vi "Zaber Manager.vi"(0 "Cmd":string="192.168.33.1", 1 "Action":T1=enum."Init", 5 "Value":dbl, 7 "File Path":path, 11 "error in (no error)":errorcluster) -> (4 "Response":string, 6 "Connected":bool, 8 "Position(um)":dbl, 10 "Position(cnts)":i64, 13 "Success":bool, 14 "Timeout":bool, 15 "error out":errorcluster)   [LabVIEW 2020]
uses:
  Mot Stage Mngr.ctl
  Lib/Serial/Find Device Protocols.ctl
  Hardware Globals.vi
  Zaber/Zaber A Series.lvlib
  Lib/Utilities.lvlib
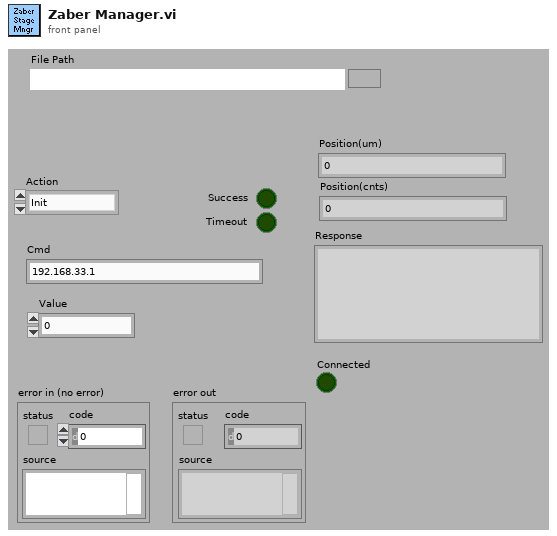
[diagram p1: front panel]
types:
  T1 = typedef "Mot Stage Mngr.ctl" = enum16{"Connect", "Init", "Status", "Send Cmd", "Current Pos", "Set Accel", "Set Max Vel", "Home", "Rel Move", "Abs Move", "Close"}
  T2 = typedef "Find Device Protocols.ctl" = enum16{"Init", "RS232(no baud)", "RS232", "RS485", "USB", "GPIB", "Ethernet"}
  T3 = enum16{"Init", "Reset", "Read", "Update", "Close"}
  T4 = cluster{"negative limit switch":bool, "positive limit switch":bool, "home switch":bool, "position marker":bool, "device enable":bool, "quick stop":bool, "general purpose J":bool, "general purpose I":bool, "general purpose H":bool, "general purpose G":bool, "general purpose F":bool, "general purpose E":bool, "general purpose D":bool, "general purpose C":bool, "general purpose B":bool, "general purpose A":bool}
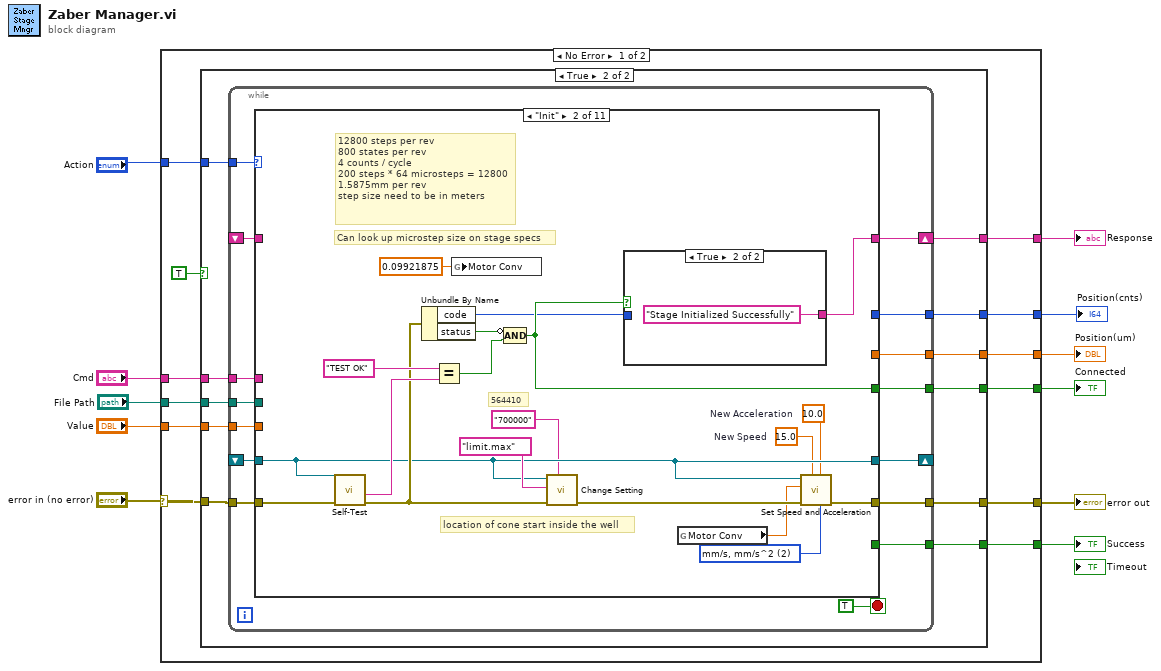
[diagram p0: block diagram]
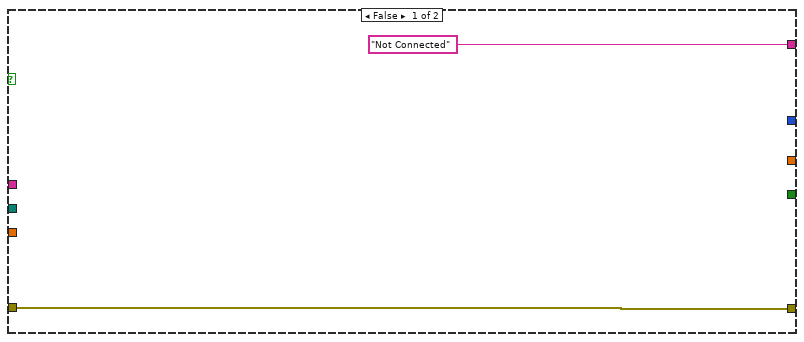
[diagram p2: hidden frame]
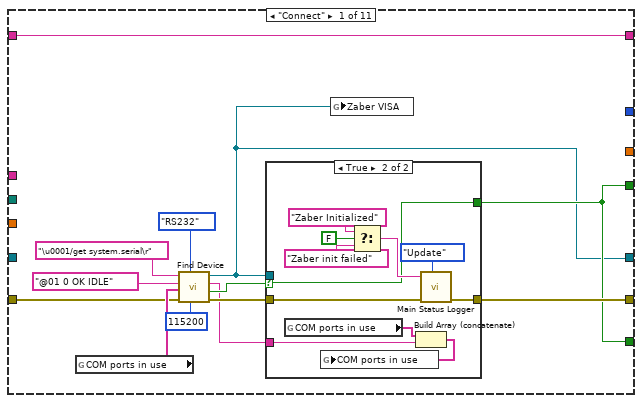
[diagram p3: hidden frame]
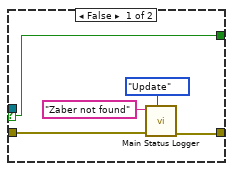
[diagram p4: hidden frame]
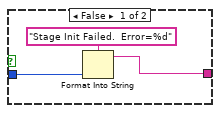
[diagram p5: hidden frame]
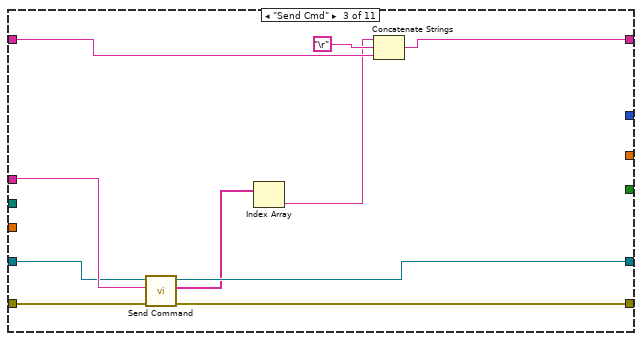
[diagram p6: hidden frame]
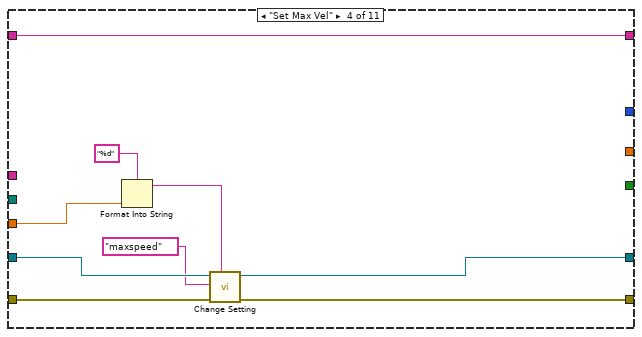
[diagram p7: hidden frame]
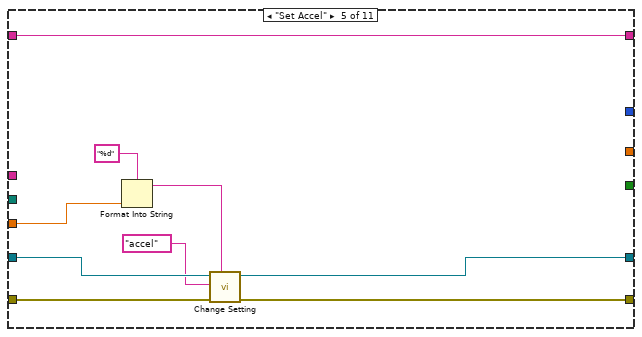
[diagram p8: hidden frame]
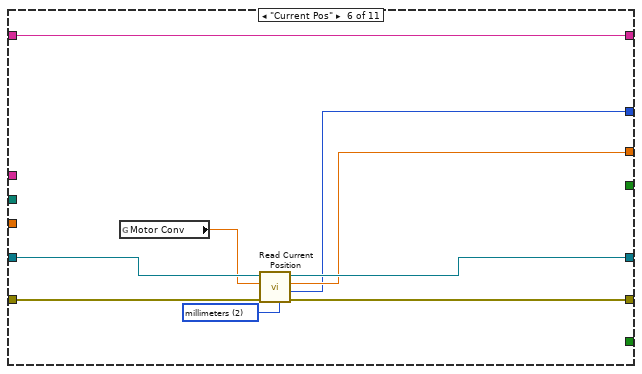
[diagram p9: hidden frame]
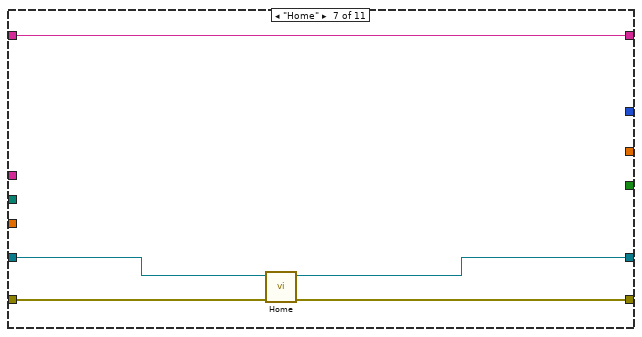
[diagram p10: hidden frame]
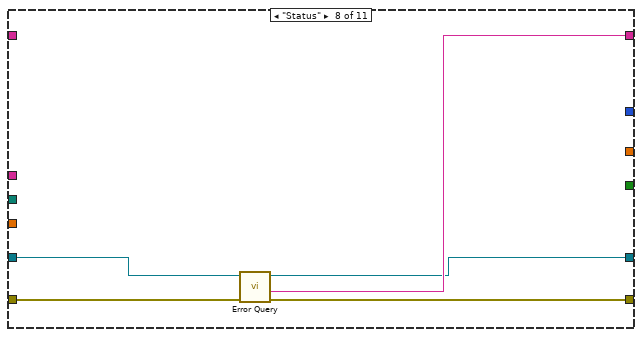
[diagram p11: hidden frame]
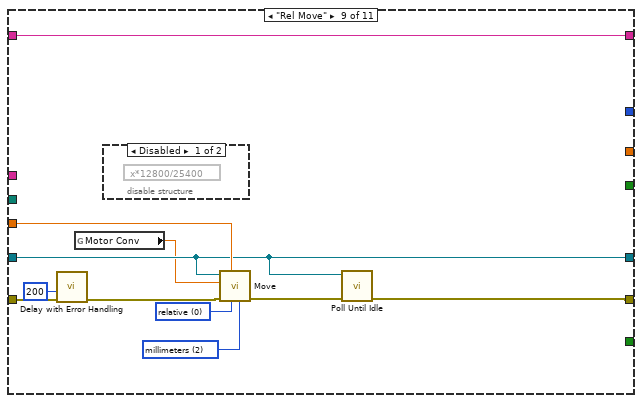
[diagram p12: hidden frame]
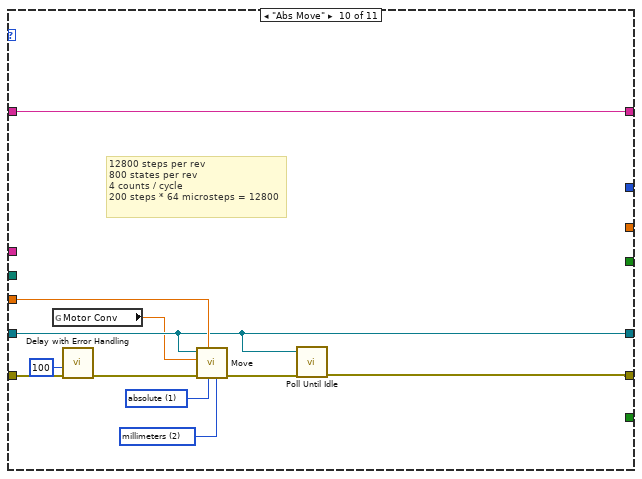
[diagram p14: hidden frame]
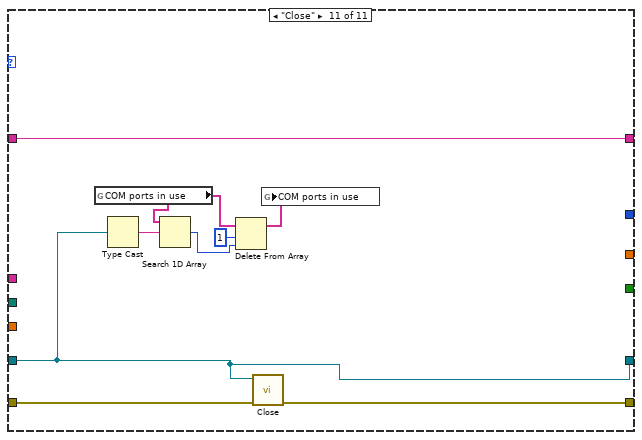
[diagram p15: hidden frame]
diagram:
  n1 = case shown="No Error" "error in (no error)" {
    selector: "error in (no error)" -> [w23 w183]
    tunnel: [w22 w183] -> w10
    tunnel: "Action" -> [w21 _]
    tunnel: "Cmd" -> [w20 _]
    tunnel: "Value" -> [w19 _]
    tunnel: [w18 "Error" ("Response")] -> w6
    tunnel: [w17 _] -> w5
    tunnel: [w15 _] -> w4
    tunnel: [w14 _] -> w3
    tunnel: "File Path" -> [w13 _]
    tunnel: [w12 _] -> w1
    frame No Error {
      n2 = case shown="True" TRUE {
        tunnel: w23 -> [w25 w36]
        tunnel: [w25 w34] -> w22
        tunnel: w21 -> [_ w35]
        tunnel: w20 -> [_ w33]
        tunnel: w19 -> [_ w32]
        tunnel: ["Not Connected" ("Response") w31] -> w18
        tunnel: [_ w30] -> w17
        tunnel: [_ w29] -> w15
        tunnel: [_ w28] -> w14
        tunnel: w13 -> [_ w27]
        tunnel: [_ w26] -> w12
        frame False {
        }
        frame True {
          n3 = while {
            tunnel: w36 -> [w51]
            tunnel: w35 -> [w50]
            tunnel: [w48] -> w34
            tunnel: w33 -> [w47]
            tunnel: w32 -> [w46]
            shift-right: [w45] -> w31
            shift-left: _ -> [w44]
            tunnel: [w43] -> w30
            tunnel: [w42] -> w29
            tunnel: [w41] -> w28
            shift-right: [w40] -> _
            shift-left: _ -> [w39]
            tunnel: w27 -> [w38]
            tunnel: [w37] -> w26
            stop <- TRUE stop-if-true
            n4 = case shown="\"Init\"" w50 {
              tunnel: w51 -> [w56 w94 w113 w122 w131 w139 w144 w150 w156 w167 w180]
              tunnel: [w55 w95 w110 w121 w130 w138 w143 w148 w152 w163 w179] -> w48
              tunnel: w47 -> [_ _ w108 _ _ _ _ _ _ _ _]
              tunnel: w46 -> [_ _ _ w116 w125 _ _ _ w155 w166 _]
              tunnel: [w54 w99 w111 w117 w126 w140 w145 w149 w161 w172 w181] -> w45
              tunnel: w44 -> [w54 _ w109 w117 w126 w140 w145 _ w161 w172 w181]
              tunnel: [w53 w97 _ _ _ _ _ _ _ _ _] -> w43
              tunnel: [_ _ _ _ _ w134 _ _ _ _ _] -> w42
              tunnel: [w53 _ _ _ _ _ _ _ _ _ _] -> w41
              tunnel: [w52 w87 w106 w119 w128 w136 w141 w147 w153 w164 w173] -> w40
              tunnel: w39 -> [_ w87 w107 w120 w129 w137 w142 w146 w153 w164 w173]
              tunnel: w38 -> [_ _ _ _ _ _ _ _ _ _ _]
              tunnel: [_ _ _ _ _ w132 _ _ _ _ _] -> w37
              frame "Connect" {
                n5 = global read "Hardware Globals.vi" "COM ports in use"() -> (w58:string[])
                n6 = call "Find Device.vi"("Baud Rate"=u32 115200, "Device Type"=Find_Device_Protocols."RS232", "error in (no error)"=w56, "Ports in Use"=w58, "ID Response"="@01 0 OK IDLE", "ID String"="\u0001/get system.serial\r") -> ("error out"=w64:errorcluster, "Device Found"=w62:bool, "device ID"=w59:string, "VISA resource name out"=w52:refnum<visa-resource-name>)  [unwired: 1 in, 1 out]
                n7 = case shown="True" w62 {
                  selector: w62 -> [w69 w71]
                  tunnel: [w66 w76] -> w55
                  tunnel: w64 -> [w67 w72]
                  tunnel: [w69 w71] -> w53
                  tunnel: w52 -> [_ _]
                  tunnel: w59 -> [_ w73]
                  frame False {
                    n8 = call "Main Status Logger.vi"("Action"=T3."Update", "error in"=w67, "Input String"="Zaber not found") -> ("error out"=w66:errorcluster)  [unwired: 7 in, 1 out]
                  }
                  frame True {
                    n9 = global read "Hardware Globals.vi" "COM ports in use"() -> (w75:string[])
                    n10 = Select(t="Zaber Initialized" ("ID Response"), s=FALSE, f="Zaber init failed" ("ID Response")) -> (s? t:f=w77:string)
                    n11 = Build Array (concatenate)(w75, w73) -> (w74:string[])
                    n12 = global write "Hardware Globals.vi" "COM ports in use"(w74) -> ()
                    n13 = call "Main Status Logger.vi"("Action"=T3."Update", "error in"=w72, "Input String"=w77) -> ("error out"=w76:errorcluster)  [unwired: 7 in, 1 out]
                  }
                }
                n14 = global write "Hardware Globals.vi" "Zaber VISA"(w52) -> ()
              }
              frame "Init" {
                w81 = u16 2 items=["device units", "microns/s, microns/s^2", "mm/s, mm/s^2", "inches/s, inches/s^2", "degrees/s, degrees/s^2"] ("Units (0: data)")
                w84 = 10.0  # New Acceleration
                w83 = 15.0  # New Speed
                (unwired) cluster{dbl, "Voltage":dbl}[][] []
                # "Can look up microstep size on stage specs"
                # "564410"
                # "location of cone start inside the well"
                # "12800 steps per rev\n800 states per rev\n4 counts / cycle\n200 steps * 64 microsteps = 12800\n1.5875mm per rev\nstep size need to be in meters"
                n15 = call "Self-Test.vi"("error in (no error)"=w94, "VISA resource name"=w87) -> ("error out"=w89:errorcluster, "Self-Test Result Message"=w93:string)  [unwired: 7 in, 1 out]
                n16 = Unbundle By Name(w89) -> ("code"=w96:i32, "status"=w98:bool)
                n17 = Equal?(x="TEST OK", y=w93) -> (x = y?=w91:bool)
                n18 = global write "Hardware Globals.vi" "Motor Conv"(0.09921875 ("Motor Conv")) -> ()
                n19 = Compound Arithmetic op=AND(invert w98, w91) -> (w97:bool)
                n20 = call "Change Setting.vi"("Data"="700000", "error in (no error)"=w89, "Setting"="limit.max" ("All Settings (Access Level 2)"), "VISA resource name"=w87) -> ("error out"=w88:errorcluster)  [unwired: 6 in, 1 out]
                n21 = case shown="True" w97 {
                  tunnel: w96 -> [w102 _]
                  tunnel: [w100 "Stage Initialized Successfully" ("Response")] -> w99
                  frame False {
                    n22 = Format Into String(format string="Stage Init Failed.  Error=%d", w102) -> (resulting string=w100:string)  [unwired: 2 in, 1 out]
                  }
                  frame True {
                  }
                }
                n23 = global read "Hardware Globals.vi" "Motor Conv"() -> (w82:dbl)
                n24 = call "Set Speed and Acceleration.vi"("Units (0: data)"=w81, "New Acceleration (0)"=w84, "New Speed (0)"=w83, "error in (no error)"=w88, "Microstep Size (0)"=w82, "VISA resource name"=w87) -> ("error out"=w95:errorcluster)  [unwired: 4 in, 1 out]
              }
              frame "Send Cmd" {
                n25 = call "Send Command.vi"("error in (no error)"=w113, "Command"=w108, "VISA resource name"=w107) -> ("error out"=w110:errorcluster, "Response String Array"=w105:string[], "VISA resource name out"=w106:refnum<visa-resource-name>)  [unwired: 3 in, 3 out]
                n26 = Index Array(array=w105) -> (element=w104:string)  [unwired: 1 in]
                n27 = Concatenate Strings(w104, "\r", w109) -> (w111:string)
              }
              frame "Set Max Vel" {
                n28 = Format Into String(format string="%d", w116) -> (resulting string=w114:string)  [unwired: 2 in, 1 out]
                n29 = call "Change Setting.vi"("Data"=w114, "error in (no error)"=w122, "Setting"="maxspeed" ("All Settings (Access Level 2)"), "VISA resource name"=w120) -> ("error out"=w121:errorcluster, "VISA resource name out"=w119:refnum<visa-resource-name>)  [unwired: 6 in]
              }
              frame "Set Accel" {
                n30 = Format Into String(format string="%d", w125) -> (resulting string=w123:string)  [unwired: 2 in, 1 out]
                n31 = call "Change Setting.vi"("Data"=w123, "error in (no error)"=w131, "Setting"="accel" ("All Settings (Access Level 2)"), "VISA resource name"=w129) -> ("error out"=w130:errorcluster, "VISA resource name out"=w128:refnum<visa-resource-name>)  [unwired: 6 in]
              }
              frame "Current Pos" {
                w135 = u16 2 items=["microsteps", "microns", "millimeters", "inches"] ("Units (0: microsteps)")
                n32 = global read "Hardware Globals.vi" "Motor Conv"() -> (w133:dbl)
                n33 = call "Read Current Position.vi"("Units (0: microsteps)"=w135, "error in (no error)"=w139, "Microstep Size (0)"=w133, "VISA resource name"=w137) -> ("error out"=w138:errorcluster, "Position cnts"=w132:i64, "Position"=w134:dbl, "VISA resource name out"=w136:refnum<visa-resource-name>)  [unwired: 4 in]
              }
              frame "Home" {
                n34 = call "Home.vi"("error in (no error)"=w144, "VISA resource name"=w142) -> ("error out"=w143:errorcluster, "VISA resource name out"=w141:refnum<visa-resource-name>)  [unwired: 8 in]
              }
              frame "Status" {
                n35 = call "Error Query.vi"("error in (no error)"=w150, "VISA resource name"=w146) -> ("error out"=w148:errorcluster, "Error Message"=w149:string, "VISA resource name out"=w147:refnum<visa-resource-name>)  [unwired: 6 in, 1 out]
              }
              frame "Rel Move" {
                w159 = u16 2 items=["microsteps", "microns", "millimeters", "inches"] ("Units (0: microsteps)")
                w160 = u16 0 items=["relative", "absolute"] ("Movement Type (0: relative)")
                n36 = call "Delay with Error Handling.vi"("error in (no error)"=w156, "Delay (ms)"=u32 200) -> ("error out"=w158:errorcluster)  [unwired: 9 in]
                n37 = global read "Hardware Globals.vi" "Motor Conv"() -> (w151:dbl)
                n38 = disable-structure shown="Disabled" {
                  frame Disabled {
                    n39 = expression code="x*12800/25400"() -> ()  [unwired: 1 in, 1 out]
                  }
                  frame Enabled {
                  }
                }
                n40 = call "Move.vi"("Units (0: microsteps)"=w159, "Movement Type (0: relative)"=w160, "Move Distance (0)"=w155, "error in (no error)"=w158, "Microstep Size (0)"=w151, "VISA resource name"=w153) -> ("error out"=w154:errorcluster)  [unwired: 4 in, 1 out]
                n41 = call "Poll Until Idle.vi"("error in (no error)"=w154, "VISA resource name"=w153) -> ("error out"=w152:errorcluster)  [unwired: 8 in, 1 out]
              }
              frame "Abs Move" {
                w170 = u16 2 items=["microsteps", "microns", "millimeters", "inches"] ("Units (0: microsteps)")
                w171 = u16 1 items=["relative", "absolute"] ("Movement Type (0: relative)")
                # "12800 steps per rev\n800 states per rev\n4 counts / cycle\n200 steps * 64 microsteps = 12800"
                n42 = global read "Hardware Globals.vi" "Motor Conv"() -> (w162:dbl)
                n43 = call "Delay with Error Handling.vi"("error in (no error)"=w167, "Delay (ms)"=u32 100) -> ("error out"=w168:errorcluster)  [unwired: 9 in]
                n44 = call "Move.vi"("Units (0: microsteps)"=w170, "Movement Type (0: relative)"=w171, "Move Distance (0)"=w166, "error in (no error)"=w168, "Microstep Size (0)"=w162, "VISA resource name"=w164) -> ("error out"=w165:errorcluster)  [unwired: 4 in, 1 out]
                n45 = call "Poll Until Idle.vi"("error in (no error)"=w165, "VISA resource name"=w164) -> ("error out"=w163:errorcluster)  [unwired: 8 in, 1 out]
              }
              frame "Close" {
                (unwired) cluster{"Elapsed Time(s)":dbl, "mean":dbl}[] []
                n46 = global read "Hardware Globals.vi" "COM ports in use"() -> (w177:string[])
                n47 = Type Cast(x=w173) -> (*(type *) &x=w178:string)  [unwired: 1 in]
                n48 = Search 1D Array(1D array=w177, element=w178) -> (index of element=w175:i32)  [unwired: 1 in]
                n49 = Delete From Array(array=w177, length=1, index=w175) -> (array with subset deleted=w174:string[])  [unwired: 1 out]
                n50 = call "Close.vi"("error in (no error)"=w180, "VISA resource name"=w173) -> ("error out"=w179:errorcluster)  [unwired: 9 in]
                n51 = global write "Hardware Globals.vi" "COM ports in use"(w174) -> ()
              }
            }
          }
        }
      }
    }
    frame Error {
      (unwired) T4 {"negative limit switch"=FALSE, "positive limit switch"=FALSE, "home switch"=FALSE, "position marker"=FALSE, "device enable"=FALSE, "quick stop"=FALSE, "general purpose J"=FALSE, "general purpose I"=FALSE, "general purpose H"=FALSE, "general purpose G"=FALSE, "general purpose F"=FALSE, "general purpose E"=FALSE, "general purpose D"=FALSE, "general purpose C"=FALSE, "general purpose B"=FALSE, "general purpose A"=FALSE} ("digital inputs")
    }
  }
  "error out" <- w10
  "Response" <- w6
  "Connected" <- w5
  "Position(um)" <- w4
  "Success" <- w3
  "Position(cnts)" <- w1
